vi "RT Tags.vi"() -> ()   [LabVIEW 2014]
panel:
  out "Low Memory":bool
  out "High CPU Usage":bool
  out "pH Exceed?":bool
  out "Temp Exceed?":bool
  out "Live Data?":bool
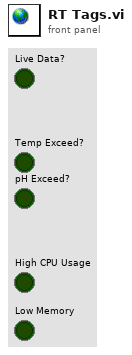
[diagram p1: front panel]
diagram:
